vi "load_current_session.vi"(3 "ListOfFiducialsPrev":T1[](array[typedef]), 4 "Current Session Information":T2={"CollectionOfPoints"=[], "Instrument"=enum."Unknown", "CollectionFile"=path "kfaj;ldkfja;f", "Session Name/ID"="", "SessionNotes"=""}, 5 "TopLevelDataFilePath":path, 6 "just a file":path) -> (0 "ListOfFiducials":T1[](array[typedef]), 1 "Fiducial Count":u32[](array[colorbox])=[3071, 3071, 3071], 2 "Sample Set":T2)   [LabVIEW 2011]
uses:
  cm2nm_sample_set.ctl
  cm2nm_coordinate_information_v2.ctl
  Instrument_type_enum_v2.ctl
  Fiducial_item.ctl
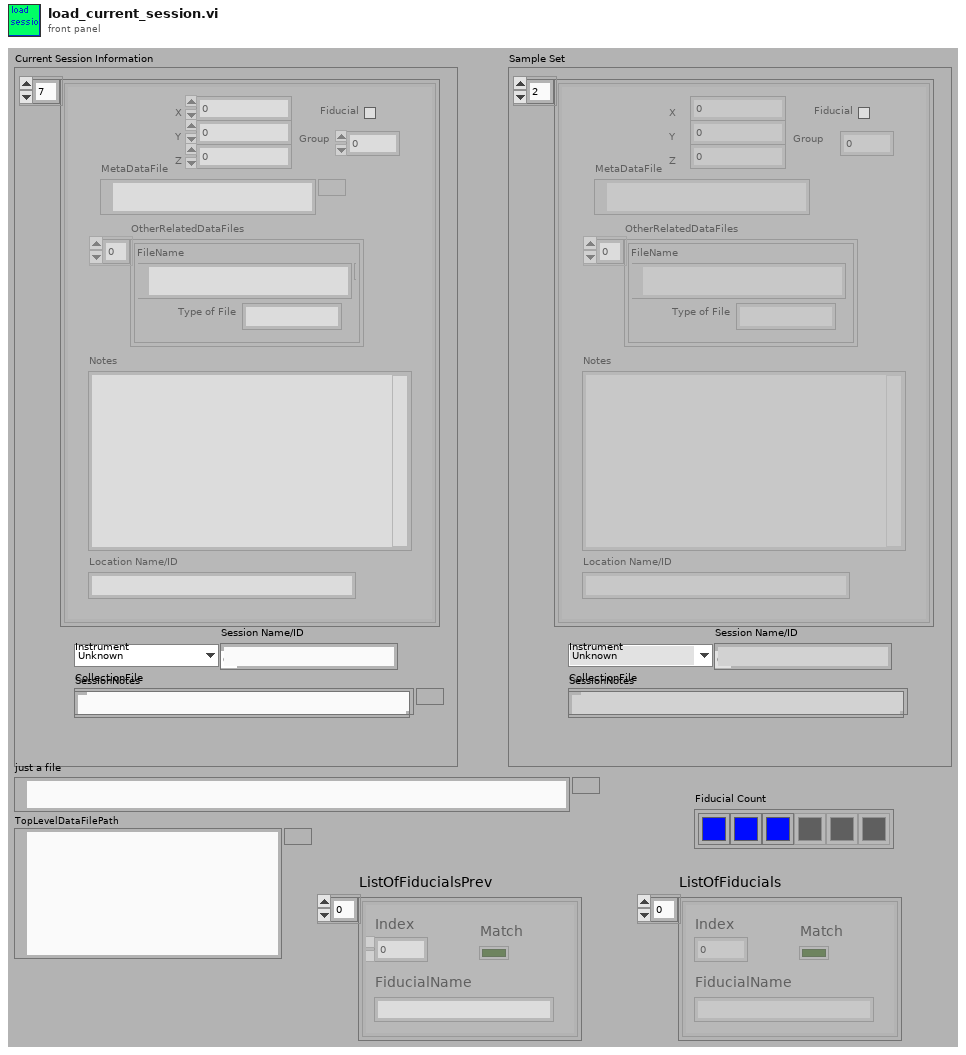
[diagram p1: front panel]
types:
  T1 = typedef "Fiducial_item.ctl" = cluster{"Index":u32, "FiducialName":string, "Match":bool}
  T2 = typedef "cm2nm_sample_set.ctl" = cluster{"CollectionOfPoints":T3[], "Instrument":T4, "CollectionFile":path, "Session Name/ID":string, "SessionNotes":string}
  T3 = typedef "cm2nm_coordinate_information_v2.ctl" = cluster{"MetaDataFile":path, "X":dbl, "Y":dbl, "Z":dbl, "Group":i32, "Rotation":dbl[unit], "Fiducial":bool, "Magnification":dbl, "Working_Distance":dbl, "Notes":string, "Location Name/ID":string, "OtherRelatedDataFiles":cluster{"Type of File":string, "FileName":path}[], "Available":bool}
  T4 = typedef "Instrument_type_enum_v2.ctl" = enum16{"Unknown", "Philips FEI SEM IRC", "JEOL 7000F EML_MFC", "MXRD MFC", "JEOL_EPMA"}
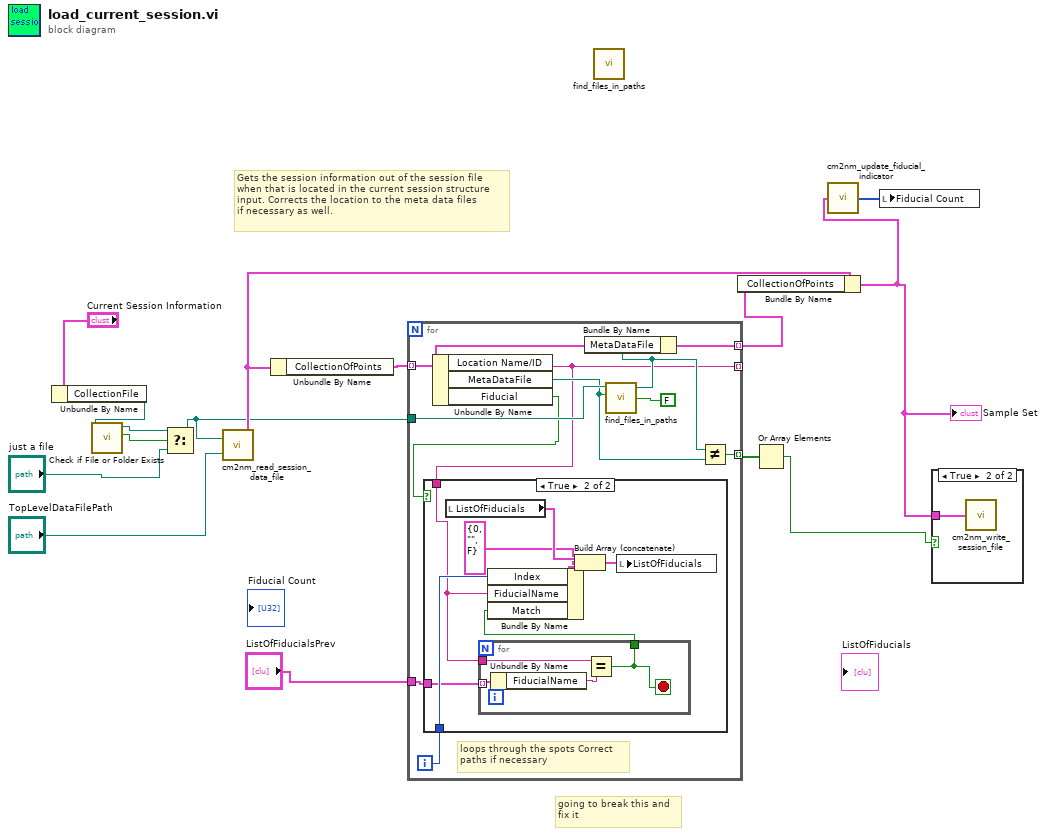
[diagram p0: block diagram]
diagram:
  # "going to break this and\nfix it"
  # "Gets the session information out of the session file\nwhen that is located in the current session structure\ninput. Corrects the location to the meta data files\nif necessary as well."
  n1 = Unbundle By Name("Current Session Information") -> ("CollectionFile"=w7:path)
  n2 = call <vilib>:"Check if File or Folder Exists.vi"("path"=w7) -> ("file or folder exists?"=w4:bool, "dup path"=w5:path)  [unwired: 8 in, 1 out]
  n3 = Select(t=w5, s=w4, f="just a file") -> (s? t:f=w6:path)
  n4 = call "cm2nm_read_session_data_file.vi"("TopLevelDataFilePath"="TopLevelDataFilePath", "Session_data_base"=w6) -> ("Session Information"=w14:T2)  [unwired: 1 in]
  n5 = Unbundle By Name(w14) -> ("CollectionOfPoints"=w15:T3[])
  n6 = for {
    tunnel: w15 -> [w25] mode=indexing
    tunnel: [w17] -> _ mode=indexing
    tunnel: w6 -> [w26]
    tunnel: [w24] -> w13 mode=indexing
    tunnel: [w20] -> w12 mode=indexing
    tunnel: "ListOfFiducialsPrev" -> [w16]
    i -> [w18]
    # "loops through the spots Correct\npaths if necessary"
    n7 = Unbundle By Name(w25) -> ("Location Name/ID"=w17:string, "MetaDataFile"=w21:path, "Fiducial"=w19:bool)
    n8 = case shown="True" w19 {
      tunnel: w18 -> [_ w30]
      tunnel: w17 -> [_ w28]
      tunnel: w16 -> [_ w29]
      frame False {
      }
      frame True {
        n9 = local read "ListOfFiducials"() -> (w33:T1[])
        n10 = for {
          tunnel: w29 -> [w37] mode=indexing
          tunnel: w28 -> [w38]
          tunnel: [w35] -> w27
          stop <- w35 stop-if-true
          n11 = Unbundle By Name(w37) -> ("FiducialName"=w36:string)
          n12 = Equal?(x=w38, y=w36) -> (x = y?=w35:bool)
        }
        n13 = Bundle By Name(cluster=T1 {"Index"=0, "FiducialName"="", "Match"=FALSE} ("element"), "Index"=w30, "FiducialName"=w28, "Match"=w27) -> (w32:T1)
        n14 = Build Array (concatenate)(w33, w32) -> (w34:T1[])
        n15 = local write "ListOfFiducials"(w34) -> ()
      }
    }
    n16 = call "find_files_in_paths.vi"("TopLevelDataFilePath"=w26, "File2Find"=w21, "PromptFormissingFile"=FALSE) -> ("Path"=w22:path)  [unwired: 3 in, 1 out]
    n17 = Bundle By Name(cluster=w25, "MetaDataFile"=w22) -> (w24:T3)
    n18 = Not Equal?(x=w22, y=w21) -> (x != y?=w20:bool)
  }
  n19 = call "find_files_in_paths.vi"() -> ()  [unwired: 6 in, 2 out]
  n20 = Bundle By Name(cluster=w14, "CollectionOfPoints"=w13) -> (w9:T2)
  "Sample Set" <- w9
  n21 = Or Array Elements(Boolean array=w12) -> (logical OR=w8:bool)
  n22 = call "cm2nm_update_fiducial_indicator.vi"("Sample Set"=w9) -> ("Array"=w10:u32[])
  n23 = local write "Fiducial Count"(w10) -> ()
  n24 = case shown="True" w8 {
    tunnel: w9 -> [_ w39]
    frame False {
    }
    frame True {
      n25 = call "cm2nm_write_session_file.vi"("Session Information"=w39) -> ()  [unwired: 1 out]
    }
  }
